vi "CRefLabel Static Reference.vi"(4 "Type":T2, 5 "Checksum":u32) -> (1 "Created":bool, 2 "Variant CReference":T1)   [LabVIEW 2012, in "CRef.lvlib"]
uses:
  CRef.lvlib
  Core/Master Types.ctl
  Interface/CRef Variant.llb/Variant CReference.ctl
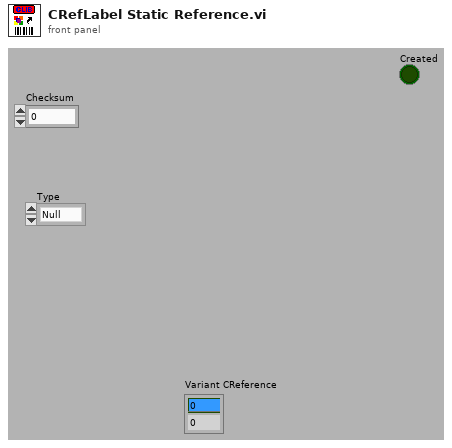
[diagram p1: front panel]
types:
  T1 = typedef "CRef.lvlib/Variant CReference.ctl" = cluster{"Generic CRef Address":u16, "Type":u8}
  T2 = typedef "CRef.lvlib/Master Types.ctl" = enum8{"Null", "Boolean", "U8", "I8", "U16", "I16", "U32", "I32", "U64", "I64", "Single", "Double", "Extended", "CSG", "CDB", "CXT", "Boolean(Def)", "U8(Def)", "I8(Def)", "U16(Def)", "I16(Def)", "U32(Def)", "I32(Def)", "Reserved Def", "Reserved Def1", "Single(Def)", "Double(Def)", "Reserved Def2", "Reserved Def3", "Reserved Def4", "Reserved Def5", "Unsigned(Def)", "Signed(Def)", "Real(Def)", "Reserved Def6", "Numeric(Def)", "String"}
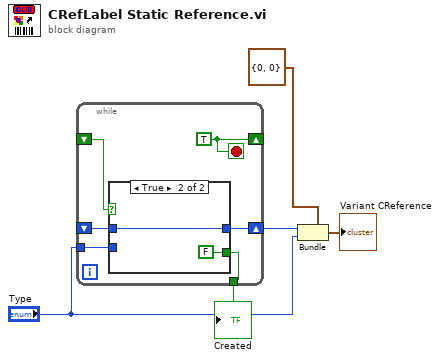
[diagram p0: block diagram]
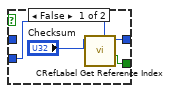
[diagram p2: hidden frame]
diagram:
  n1 = while {
    shift-right: [w11] -> w3
    shift-left: _ -> [w10]
    shift-right: [w8] -> _
    shift-left: _ -> [w9]
    tunnel: "Type" -> [w7]
    tunnel: [w6] -> w1
    stop <- w8 stop-if-true
    w8 = TRUE
    n2 = case shown="True" w9 {
      tunnel: [w15 w17] -> w11
      tunnel: w10 -> [_ w17]
      tunnel: w7 -> [w13 _]
      tunnel: [w12 FALSE ("Created")] -> w6
      frame False {
        n3 = call "CRefLabel Get Reference Index.vi"("Checksum"="Checksum", "(new) Type"=w13) -> ("Created"=w12:bool, "Address"=w15:i32)  [unwired: 8 in]
      }
      frame True {
      }
    }
  }
  "Created" <- w1
  n4 = Bundle(cluster=T1 {"Generic CRef Address"=0, "Type"=0} ("Variant CReference"), "Generic CRef Address"=w3, "Type"="Type") -> (→"Variant CReference":T1)
